vi "assemble.vi"(8 "error in (no error)":errorcluster, 11 "Table in":refnum<class "Table.lvclass">) -> (0 "error out":errorcluster, 2 "String":string="assembeld", 3 "Table out":refnum<class "Table.lvclass">)   [LabVIEW 2021, in "Table.lvclass"]
uses:
  Table.lvclass
  Furniture/Furniture.lvclass
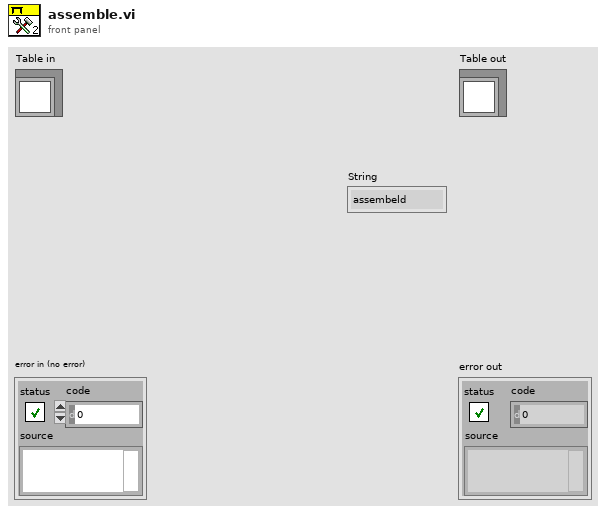
[diagram p1: front panel]
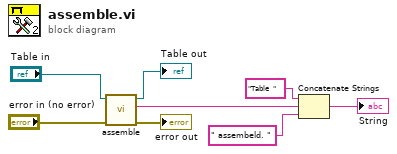
[diagram p0: block diagram]
diagram:
  n1 = call-parent "assemble.vi"("error in (no error)"="error in (no error)", "Furniture in"="Table in") -> ("error out"=→"error out":errorcluster, "String"=w1:string, "Furniture out"=→"Table out":refnum<class "Table.lvclass">)  [unwired: 7 in]
  n2 = Concatenate Strings("Table  ", w1, " assembeld. ") -> (→"String":string)
